vi "Cash Karp Global.vi"() -> ()   [LabVIEW 2018, in "NI_Gmath.lvlib"]
uses:
  NI_Gmath.lvlib
panel:
  in  "zero":dbl[](array[numeric])=[0.0, 0.0, 0.0, 0.0, 0.0, 0.0] format="%.4f"
  out "result":dbl[](array[numeric]) format="%.2f"
  out "table":i32[][](array[numeric])
  in  "c*":dbl[](array[numeric])=[0.102177372685, 0.0, 0.383907903439, 0.244592737269, 0.019321986607, 0.25] format="%.4f"
  in  "c":dbl[](array[numeric])=[0.097883597884, 0.0, 0.402576489533, 0.210437710438, 0.0, 0.289102202146] format="%.4f"
  in  "b":dbl[][](array[numeric])=[[0.0, 0.0, 0.0, 0.0, 0.0], [0.2, 0.0, 0.0, 0.0, 0.0], [0.075, 0.225, 0.0, 0.0, 0.0], [0.3, -0.9, 1.2, 0.0, 0.0], [-0.2037, 2.5, -2.592592592593, 1.296296296296, 0.0], [0.029495804398, 0.341796875, 0.041594328704, 0.400345413773, 0.061767578125]] format="%.4f"
  in  "a":dbl[](array[numeric])=[0.0, 0.2, 0.3, 0.6, 1.0, 0.875] format="%.4f"
  # "Attention: these values are constants!"
  # "operator"
  # "register1"
  # "register2"
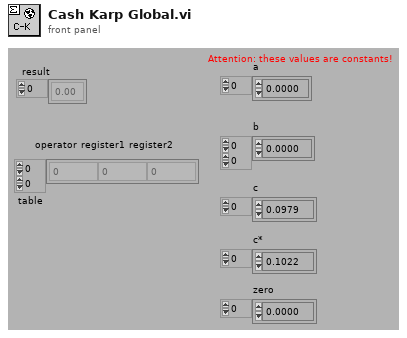
[diagram p1: front panel]
diagram:
